vi "Get Host IP.vi"(8 "error in (no error)":errorcluster, 10 "pNumberofHost":u32, 11 "pHostIP":u32) -> (0 "error out":errorcluster, 1 "function return":i32, 2 "pNumberofHost out":u32, 3 "pHostIP out":u32)   [LabVIEW 2017, in "imgAcquisiotn.lvlib"]
doc: "DLLFunction int __stdcall ImageCapGetHostIP(unsigned int* pHostIP, unsigned int* pNumberofHost);"
uses:
  imgAcquisiotn.lvlib
  lib/ImageCaptureDLL.dll
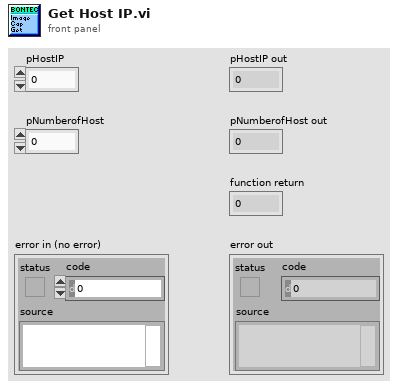
[diagram p1: front panel]
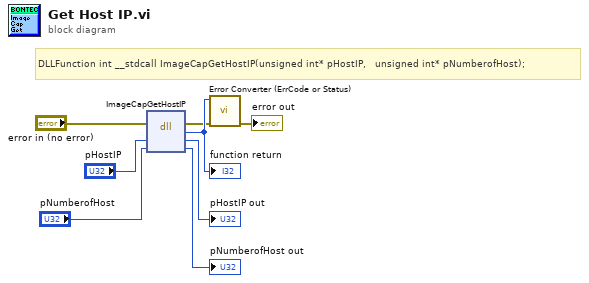
[diagram p0: block diagram]
diagram:
  # "DLLFunction int __stdcall ImageCapGetHostIP(unsigned int* pHostIP,   unsigned int* pNumberofHost);"
  n1 = dll-call lib="F:/BonTechFlatPanelLVDriver/lib/ImageCaptureDLL.*" fn="ImageCapGetHostIP"(error in="error in (no error)", "pHostIP"="pHostIP", "pNumberofHost"="pNumberofHost") -> (error out=w2:errorcluster, w8:i32, "pHostIP"=→"pHostIP out":u32, "pNumberofHost"=→"pNumberofHost out":u32)  [unwired: 2 in, 1 out]
  "function return" <- w8
  n2 = call "Error Converter (ErrCode or Status).vi"("error in (no error)"=w2, "error code"=w8) -> ("error out"=→"error out":errorcluster)  [unwired: 9 in]
